vi "Navigation_Main_derping_stuff_up 5th.vi"() -> ()   [LabVIEW 2015]
uses:
  <vilib>/myRIO/Common/Instrument Driver Framework/Utilities/typedefs/Generic FPGA Reference.ctl
  <vilib>/myRIO/Common/Instrument Driver Framework/Utilities/typedefs/myRIO v1.0 Reference.ctl
  <vilib>/myRIO/Common/Instrument Driver Framework/Utilities/typedefs/Hardware Version Enum.ctl
  <vilib>/myRIO/Common/Instrument Driver Framework/Utilities/typedefs/myRIO Generic Hardware Reference.ctl
  <vilib>/userdefined/High Color/nirio_resource_hc.ctl
  <vilib>/myRIO/Instrument Drivers/Onboard IO/PWM/typedefs/PWM Configuration.ctl
  <vilib>/myRIO/Instrument Drivers/Onboard IO/PWM/PWM.lvlib
  <vilib>/myRIO/Common/Instrument Driver Framework/myRIO v1.0/PWM/typedefs/PWM Channels Enum.ctl
  <vilib>/myRIO/Instrument Drivers/Onboard IO/PWM/typedefs/PWM Reference.ctl
  <vilib>/myRIO/Instrument Drivers/Onboard IO/PWM/vis/myRIO PWM Open.xnode
  <vilib>/myRIO/Common/Instrument Driver Framework/myRIO v1.0/PWM/vis/myRIO v1.1 Open PWM.vi
  <vilib>/rvi/interface/nirviOpenFPGA/nirviOpenFPGA.xnode
  <vilib>/myRIO/Instrument Drivers/Utilities/Utilities.lvlib
  <vilib>/rvi/interface/nirviReadWriteControl/nirviReadWriteControl.xnode
  <vilib>/rvi/interface/Simulation/niFpgaSimulationCallBeginRW.vi
  <vilib>/rvi/errors/niLvFpgaAdjustHostInterfaceError.vi
  UNCC_AST2_Master/FPGA Bitfiles/NavigationProjec_FPGATarget2_FPGAMainNavigati_PWPHW8gwDxI.lvbitx
  <vilib>/addons/control/pid/NI_PID_pid.lvlib
  <vilib>/addons/control/pid/pid.llb/PID (DBL).vi
  <vilib>/FPGAPlugInAG/myRIO-1900/niLvFpga_Open_myRIO-1900.vi
  <vilib>/rvi/interface/common/dynamic/niFpgaDynamicAddResources.vi
panel:
  out "x/y":dbl
  out "scale":dbl=1.0
  in  "x goal":dbl=20.0
  out "left":dbl
  out "right":dbl
  out "actual pwm left":dbl
  in  "stop 3":bool
  out "left pwm":dbl(graph)
  out "dt out (s) left":dbl format="%.3f"
  in  "output range 3":cluster{"output high":dbl, "output low":dbl}={"output high"=0.13333, "output low"=-0.13333} {"output low" format="%.6f"; "output high" format="%.5f"}
  in  "PID gains 3":T1={"proportional gain (Kc)"=0.002, "integral time (Ti, min)"=7e-07, "derivative time (Td, min)"=0.0} {"derivative time (Td, min)" format="%.8f"; "integral time (Ti, min)" format="%.8f"; "proportional gain (Kc)" format="%.8f"}
  out "desired pwm 2":dbl
  out "feedback 2":dbl
  out ".not. x? 3":bool
  out "Elapsed Time (s) 2":dbl caption="Elapsed Time (s)"
  out "x traveled 2":dbl
  out "y traveled 2":dbl
  out "avg 124":dbl
  out "avg 457":dbl
  out "psi dot 2":dbl
  out "distance traveled 2":dbl
  out "y dot 2":dbl
  out "x dot 2":dbl
  out "x position 2":dbl
  out "y position 2":dbl
  out "reset x y 2":dbl
  out "Tick Count(mSec) 2":u32 caption="Tick Count(mSec)"
  in  "start y 2":dbl=3.0
  in  "start x 2":dbl=1.0
  in  "start y":dbl=3.0
  in  "start x":dbl=1.0
  out "actual pwm right":dbl
  in  "stop 2":bool
  out "right pwm":dbl(graph)
  out "dt out (s) right":dbl format="%.3f"
  in  "output range 2":cluster{"output high":dbl, "output low":dbl}={"output high"=0.13333, "output low"=-0.13333} {"output low" format="%.6f"; "output high" format="%.5f"}
  in  "PID gains 2":T1={"proportional gain (Kc)"=0.002, "integral time (Ti, min)"=7e-07, "derivative time (Td, min)"=0.0} {"derivative time (Td, min)" format="%.8f"; "integral time (Ti, min)" format="%.8f"; "proportional gain (Kc)" format="%.8f"}
  out "desired pwm":dbl
  out "feedback right":dbl
  out ".not. x? 2":bool
  out "Elapsed Time (s)":dbl
  out "LF Rot Velocity (rot/s)":dbl
  out "LM Rot Velocity (rot/s)":dbl
  out "LR Rot Velocity (rot/s)":dbl
  out "RR Rot Velocity (rot/s)":dbl
  out "RM Linear Velocity (rot/s)":dbl
  out "RF Linear Velocity (rot/s)":dbl
  in  "Encoder Reset":bool
  out "SYS.SELECTA":u8 format="%08b"
  out "ENC.B_c.CNTR":i32
  out "ENC.B_b.CNTR":i32
  out "ENC.B_a.CNTR":i32
  out "ENC.A_c.CNTR":i32
  out "ENC.A_b.CNTR":i32
  out "ENC.A_a.CNTR":i32
  in  "R Min Linear Velocity (ft/s)":dbl=-2.0 format="%#_13g"
  in  "R Max Linear Velocity (ft/s)":dbl=2.0 format="%#_13g"
  in  "L Min Linear Velocity (ft/s)":dbl=-2.0 format="%#_13g"
  in  "L Max Linear Velocity (ft/s)":dbl=2.0 format="%#_13g"
  out "Current Rot Velocity (rot/s)":T2(graph)
  # "Motor Control Parameters"
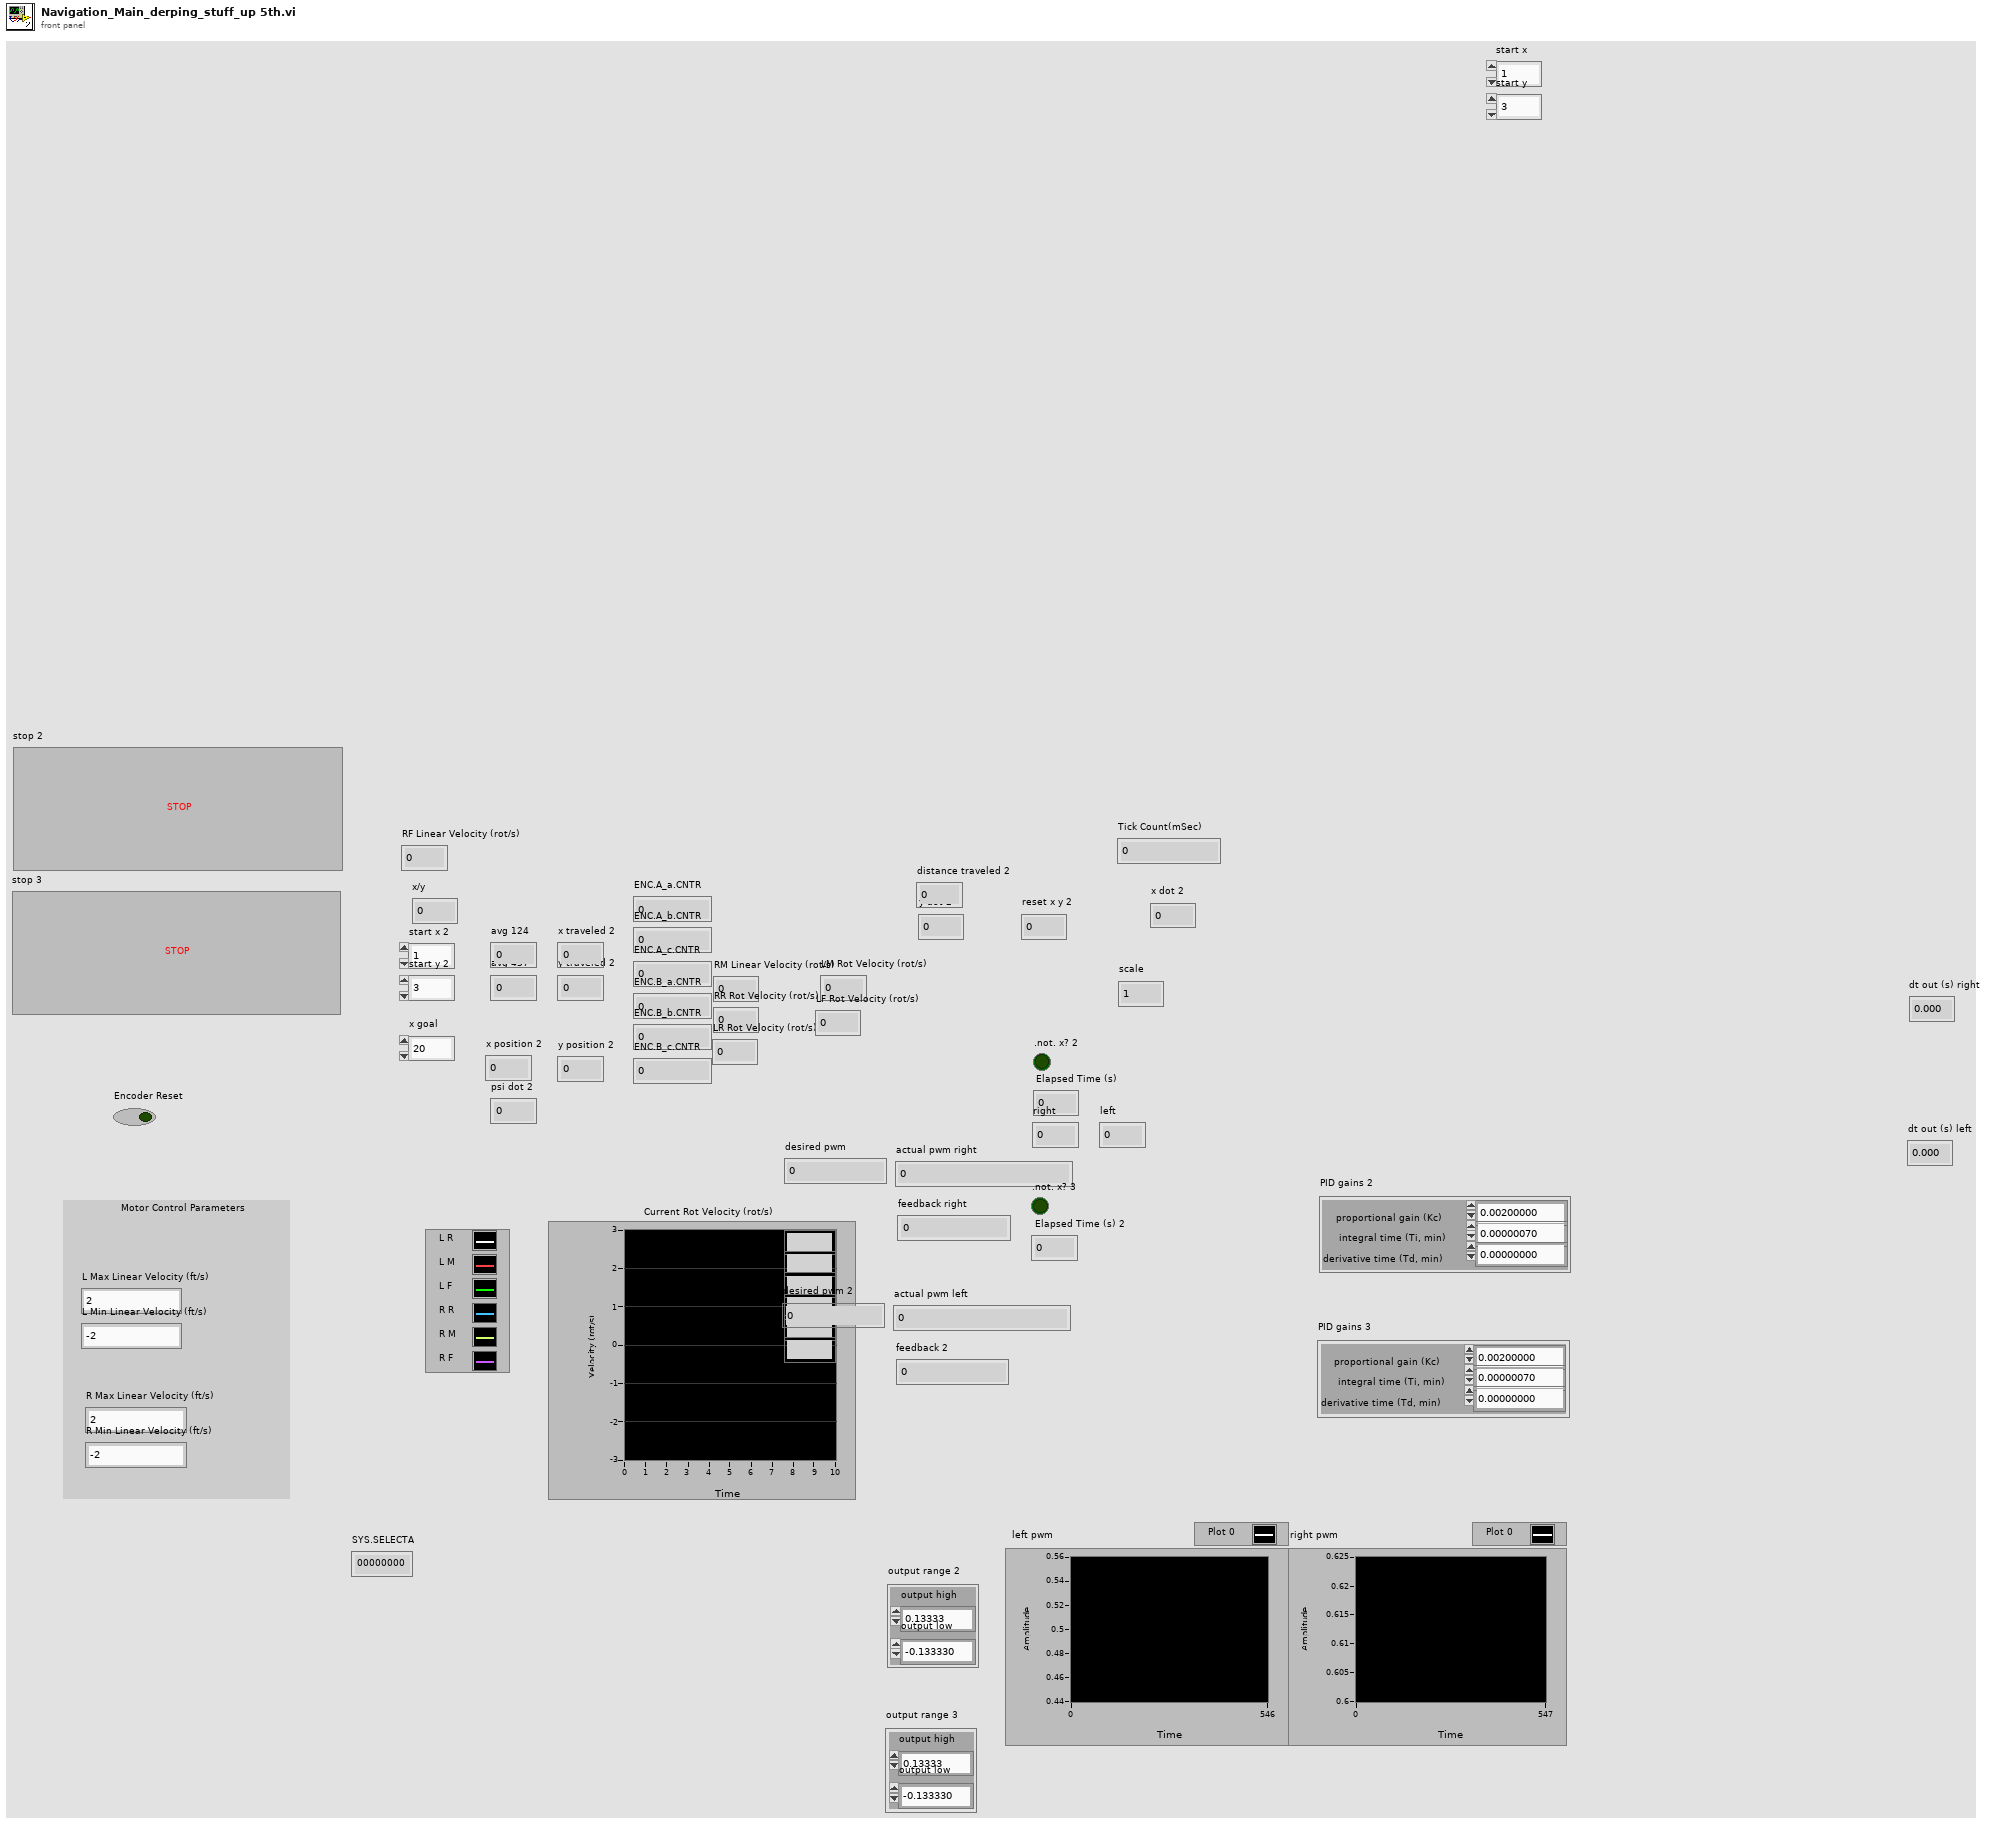
[diagram p1: front panel]
types:
  T1 = cluster{"proportional gain (Kc)":dbl, "integral time (Ti, min)":dbl, "derivative time (Td, min)":dbl}
  T2 = cluster{"Rotational Velocity (RPS)":dbl, "Rotational Velocity (RPS)":dbl, "Rotational Velocity (RPS)":dbl, "Rotational Velocity (RPS)":dbl, "Rotational Velocity (RPS)":dbl, "Rotational Velocity (RPS)":dbl}
  T3 = typedef "nirio_resource_hc.ctl" = tag
  T4 = typedef "Hardware Version Enum.ctl" = enum16{"Unknown", "myRIO-1900", "myRIO-1950", "roboRIO"}
  T5 = typedef "PWM.lvlib/PWM Reference.ctl" = cluster{"myRIO Reference":T6, "PWM Channels Enum":T9, "PWM Configuration":T10}
  T6 = typedef "myRIO Generic Hardware Reference.ctl" = cluster{"myRIO Model":T4, "myRIO Hardware Reference":T7}
  T7 = typedef "myRIO v1.0 Reference.ctl" = cluster{"Generic FPGA Reference":T8, "Allow multiple opens":bool}
  T8 = typedef "Generic FPGA Reference.ctl" = refnum<k20>
  T9 = typedef "PWM Channels Enum.ctl" = enum16{"Not Connected", "C/PWM0", "C/PWM1", "A/PWM0", "A/PWM1", "A/PWM2", "B/PWM0", "B/PWM1", "B/PWM2", "PWM/PWM0", "PWM/PWM1", "PWM/PWM2", "PWM/PWM3", "PWM/PWM4", "PWM/PWM5", "PWM/PWM6", "PWM/PWM7", "PWM/PWM8", "PWM/PWM9"}
  T10 = typedef "PWM.lvlib/PWM Configuration.ctl" = cluster{"Frequency":dbl, "Duty Cycle":dbl}
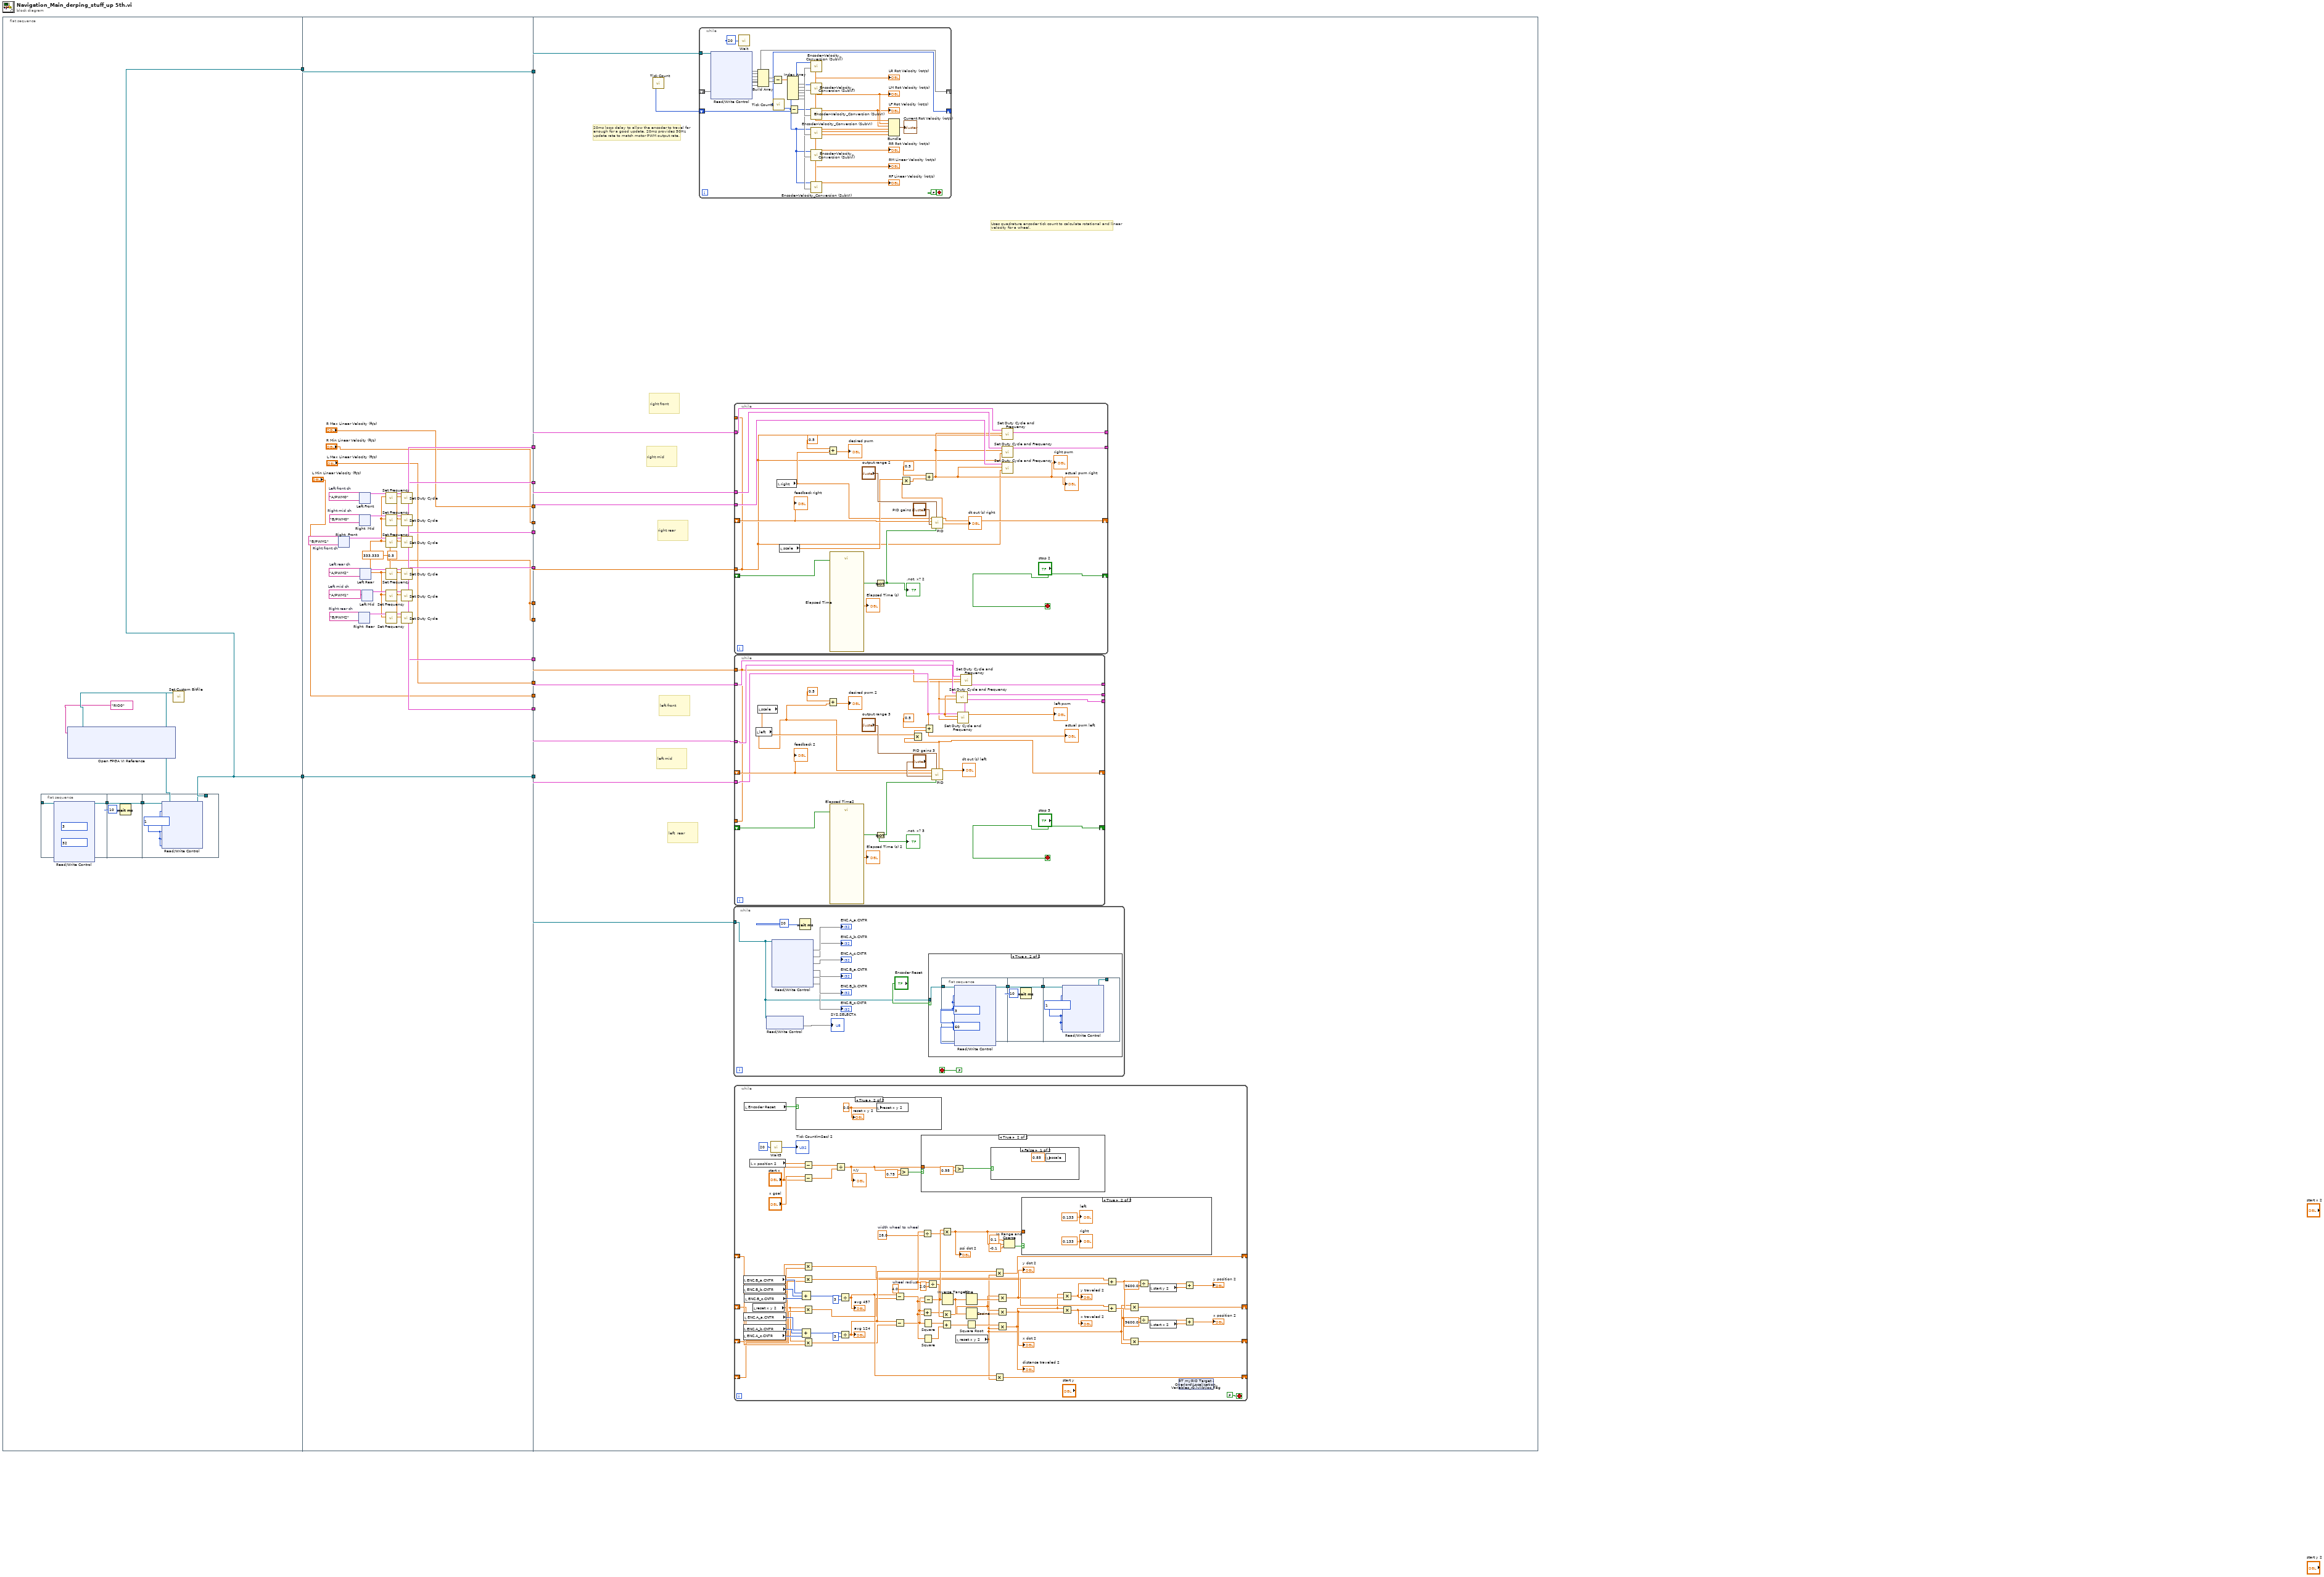
[diagram p0: block diagram]
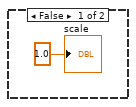
[diagram p2: hidden frame]
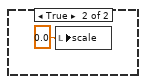
[diagram p3: hidden frame]
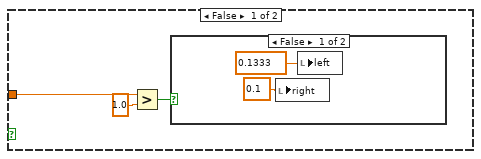
[diagram p4: hidden frame]
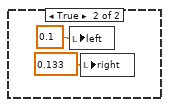
[diagram p5: hidden frame]
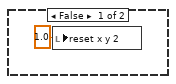
[diagram p6: hidden frame]
diagram:
  n1 = flat-sequence {
    tunnel: [w19] -> w4
    tunnel: [w19] -> w2
    tunnel: [w32] -> w16
    tunnel: [w47] -> w15
    tunnel: [w43] -> w14
    tunnel: [w42] -> w13
    tunnel: [w41] -> w12
    tunnel: [w40] -> w11
    tunnel: [w39] -> w10
    tunnel: ["L Max Linear Velocity (ft/s)"] -> w9
    tunnel: ["L Min Linear Velocity (ft/s)"] -> w8
    tunnel: ["R Max Linear Velocity (ft/s)"] -> w7
    tunnel: ["R Min Linear Velocity (ft/s)"] -> w6
    tunnel: [w34] -> w5
    tunnel: w4 -> [w33]
    tunnel: [w33] -> w3
    tunnel: w2 -> [w34]
    tunnel: [w32] -> w1
    tunnel: w16 -> [_]
    tunnel: w15 -> [w160]
    tunnel: w14 -> [w166]
    tunnel: w13 -> [w162]
    tunnel: w12 -> [w163]
    tunnel: w11 -> [w161]
    tunnel: w10 -> [w165]
    tunnel: w9 -> [_]
    tunnel: w8 -> [_]
    tunnel: w7 -> [_]
    tunnel: w6 -> [_]
    tunnel: w5 -> [w168]
    tunnel: w3 -> [w167]
    tunnel: w1 -> [w164]
    frame #0 {
      n2 = flat-sequence {
        tunnel: w20 -> [w25]
        tunnel: [w23] -> w22
        tunnel: w22 -> [w27]
        tunnel: [w27] -> w21
        tunnel: w21 -> [w30]
        tunnel: [w29] -> w19
        frame #0 {
          w24 = u8 32 ("SYS.SELECTA")
          w26 = u8 3 ("ENC.B_c.CNFG")
          n3 = xnode "Read/Write Control"("FPGA VI Reference In"=w25, "ENC.A_a.CNFG"=w26, "ENC.A_b.CNFG"=w26, "ENC.A_c.CNFG"=w26, "ENC.B_a.CNFG"=w26, "ENC.B_b.CNFG"=w26, "ENC.B_c.CNFG"=w26, "SYS.SELECTA"=w24, "SYS.SELECTB"=w24) -> ("FPGA VI Reference Out"=w23:refnum<k20>)  [unwired: 1 in, 1 out]
        }
        frame #1 {
          n4 = Wait (ms)(milliseconds to wait=u32 10) -> ()  [unwired: 1 out]
        }
        frame #2 {
          w31 = u8 1 ("ENC.B_c.CNFG")
          n5 = xnode "Read/Write Control"("FPGA VI Reference In"=w30, "ENC.A_a.CNFG"=w31, "ENC.A_b.CNFG"=w31, "ENC.A_c.CNFG"=w31, "ENC.B_a.CNFG"=w31, "ENC.B_b.CNFG"=w31, "ENC.B_c.CNFG"=w31) -> ("FPGA VI Reference Out"=w29:refnum<k20>)  [unwired: 1 in, 1 out]
        }
      }
      n6 = xnode "Open FPGA VI Reference"("resource name"=tag "RIO0") -> ("FPGA VI Reference Out"=w18:refnum<k20>)  [unwired: 1 in, 1 out]
      n7 = call <vilib>:"Set Custom Bitfile.vi"("Custom FPGA Reference In"=w18) -> ("Custom FPGA Reference Out"=w20:refnum<k20>)  [unwired: 9 in, 1 out]
    }
    frame #1 {
      w44 = 0.5 ("Duty Cycle")
      w32 = 333.333 ("Frequency [Hz]")
      w58 = tag "B/PWM2"  # Right rear ch
      w59 = tag "B/PWM0"  # Right mid ch
      w60 = tag "B/PWM1"  # Right front ch
      w61 = tag "A/PWM2"  # Left rear ch
      w62 = tag "A/PWM1"  # Left mid ch
      w63 = tag "A/PWM0"  # Left front ch
      n8 = xnode "Right  Front"("Channel Name"=w60) -> ("PWM Ref Out"=w54:T5)  [unwired: 2 in, 1 out]
      n9 = xnode "Right  Rear"("Channel Name"=w58) -> ("PWM Ref Out"=w52:T5)  [unwired: 2 in, 1 out]
      n10 = xnode "Left Front"("Channel Name"=w63) -> ("PWM Ref Out"=w57:T5)  [unwired: 2 in, 1 out]
      n11 = xnode "Right  Mid"("Channel Name"=w59) -> ("PWM Ref Out"=w53:T5)  [unwired: 2 in, 1 out]
      n12 = xnode "Left Rear"("Channel Name"=w61) -> ("PWM Ref Out"=w55:T5)  [unwired: 2 in, 1 out]
      n13 = xnode "Left Mid"("Channel Name"=w62) -> ("PWM Ref Out"=w56:T5)  [unwired: 2 in, 1 out]
      n14 = call <vilib>:"Set Frequency.vi"("Frequency [Hz]"=w32, "PWM Ref In"=w57) -> ("PWM Ref Out"=w51:T5)  [unwired: 7 in, 1 out]
      n15 = call <vilib>:"Set Frequency.vi"("Frequency [Hz]"=w32, "PWM Ref In"=w53) -> ("PWM Ref Out"=w49:T5)  [unwired: 7 in, 1 out]
      n16 = call <vilib>:"Set Frequency.vi"("Frequency [Hz]"=w32, "PWM Ref In"=w54) -> ("PWM Ref Out"=w48:T5)  [unwired: 7 in, 1 out]
      n17 = call <vilib>:"Set Frequency.vi"("Frequency [Hz]"=w32, "PWM Ref In"=w55) -> ("PWM Ref Out"=w46:T5)  [unwired: 7 in, 1 out]
      n18 = call <vilib>:"Set Frequency.vi"("Frequency [Hz]"=w32, "PWM Ref In"=w56) -> ("PWM Ref Out"=w45:T5)  [unwired: 7 in, 1 out]
      n19 = call <vilib>:"Set Frequency.vi"("Frequency [Hz]"=w32, "PWM Ref In"=w52) -> ("PWM Ref Out"=w50:T5)  [unwired: 7 in, 1 out]
      n20 = call <vilib>:"Set Duty Cycle.vi"("Duty Cycle"=w44, "PWM Ref In"=w51) -> ("PWM Ref Out"=w39:T5)  [unwired: 7 in, 1 out]
      n21 = call <vilib>:"Set Duty Cycle.vi"("Duty Cycle"=w44, "PWM Ref In"=w49) -> ("PWM Ref Out"=w42:T5)  [unwired: 7 in, 1 out]
      n22 = call <vilib>:"Set Duty Cycle.vi"("Duty Cycle"=w44, "PWM Ref In"=w48) -> ("PWM Ref Out"=w43:T5)  [unwired: 7 in, 1 out]
      n23 = call <vilib>:"Set Duty Cycle.vi"("Duty Cycle"=w44, "PWM Ref In"=w46) -> ("PWM Ref Out"=w47:T5)  [unwired: 7 in, 1 out]
      n24 = call <vilib>:"Set Duty Cycle.vi"("Duty Cycle"=w44, "PWM Ref In"=w45) -> ("PWM Ref Out"=w40:T5)  [unwired: 7 in, 1 out]
      n25 = call <vilib>:"Set Duty Cycle.vi"("Duty Cycle"=w44, "PWM Ref In"=w50) -> ("PWM Ref Out"=w41:T5)  [unwired: 7 in, 1 out]
    }
    frame #2 {
      # "left  rear"
      # "left mid"
      # "left front"
      # "right rear"
      # "right mid"
      # "right front"
      # "Uses quadrature encoder tick count to calculate rotational and linear velocity for a wheel."
      # "20ms loop delay to allow the encoder to travel far enough for a good update. 20ms provides 50Hz update rate to match motor PWM output rate."
      n26 = call "Tick Count"() -> ("Tick Count(uSec)"=w169:u32)
      n27 = while {
        shift-right: [w349] -> _
        shift-left: _ -> [w348]
        shift-right: [w346] -> _
        shift-left: w169 -> [w345]
        tunnel: w167 -> [w356]
        stop <- FALSE stop-if-true
        n28 = xnode "Read/Write Control"("FPGA VI Reference In"=w356) -> ("ENC.A_a.CNTR"=w355, "ENC.A_b.CNTR"=w354, "ENC.A_c.CNTR"=w353, "ENC.B_a.CNTR"=w352, "ENC.B_b.CNTR"=w351, "ENC.B_c.CNTR"=w350)  [unwired: 1 in, 2 out]
        n29 = call "Wait"("Count(mSec)"=u32 20) -> ()  [unwired: 1 out]
        n30 = Build Array(w355, w354, w353, w352, w351, w350) -> (w349:void[])
        n31 = Subtract(x=w349, y=w348) -> (x-y=w347:dbl)
        n32 = call "Tick Count2"() -> ("Tick Count(uSec)"=w346:u32)
        n33 = Index Array(array=w347) -> (element #1=w344, element #2=w343, element #3=w342, element #4=w341, element #5=w340, element #6=w339)  [unwired: 6 in]
        n34 = Subtract(x=w346, y=w345) -> (x-y=w338:u32)
        n35 = call "Encoder-Velocity_Conversion (SubVI).vi"("delta  Encoder Count"=w343, "dt (uSec)"=w338) -> ("Rotational Velocity (RPS)"=w333:dbl)  [unwired: 7 in, 2 out]
        "LM Rot Velocity (rot/s)" <- w333
        n36 = call "Encoder-Velocity_Conversion (SubVI).vi"("delta  Encoder Count"=w342, "dt (uSec)"=w338) -> ("Rotational Velocity (RPS)"=w332:dbl)  [unwired: 7 in, 2 out]
        "LF Rot Velocity (rot/s)" <- w332
        n37 = call "Encoder-Velocity_Conversion (SubVI).vi"("delta  Encoder Count"=w344, "dt (uSec)"=w338) -> ("Rotational Velocity (RPS)"=w334:dbl)  [unwired: 7 in, 2 out]
        "LR Rot Velocity (rot/s)" <- w334
        n38 = call "Encoder-Velocity_Conversion (SubVI).vi"("delta  Encoder Count"=w341, "dt (uSec)"=w338) -> ("Rotational Velocity (RPS)"=w331:dbl)  [unwired: 7 in, 2 out]
        "RR Rot Velocity (rot/s)" <- w331
        n39 = call "Encoder-Velocity_Conversion (SubVI).vi"("delta  Encoder Count"=w340, "dt (uSec)"=w338) -> ("Rotational Velocity (RPS)"=w335:dbl)  [unwired: 7 in, 2 out]
        "RM Linear Velocity (rot/s)" <- w335
        n40 = call "Encoder-Velocity_Conversion (SubVI).vi"("delta  Encoder Count"=w339, "dt (uSec)"=w338) -> ("Rotational Velocity (RPS)"=w336:dbl)  [unwired: 7 in, 2 out]
        "RF Linear Velocity (rot/s)" <- w336
        n41 = Bundle("Rotational Velocity (RPS)"=w334, "Rotational Velocity (RPS)"=w333, "Rotational Velocity (RPS)"=w332, "Rotational Velocity (RPS)"=w331, "Rotational Velocity (RPS)"=w335, "Rotational Velocity (RPS)"=w336) -> (→"Current Rot Velocity (rot/s)":T2)  [unwired: 1 in]
      }
      n42 = while {
        tunnel: w168 -> [w308]
        stop <- FALSE stop-if-true
        n43 = xnode "Read/Write Control"("FPGA VI Reference In"=w308) -> ("SYS.SELECTA"=→"SYS.SELECTA")  [unwired: 1 in, 2 out]
        n44 = xnode "Read/Write Control"("FPGA VI Reference In"=w308) -> ("ENC.A_a.CNTR"=→"ENC.A_a.CNTR", "ENC.A_b.CNTR"=→"ENC.A_b.CNTR", "ENC.A_c.CNTR"=→"ENC.A_c.CNTR", "ENC.B_a.CNTR"=→"ENC.B_a.CNTR", "ENC.B_b.CNTR"=→"ENC.B_b.CNTR", "ENC.B_c.CNTR"=→"ENC.B_c.CNTR")  [unwired: 1 in, 2 out]
        n45 = Wait (ms)(milliseconds to wait=u32 20) -> ()  [unwired: 1 out]
        n46 = case shown="True" "Encoder Reset" {
          tunnel: w308 -> [_ w319]
          frame False {
          }
          frame True {
            n47 = flat-sequence {
              tunnel: w319 -> [w324]
              tunnel: [w322] -> w321
              tunnel: w321 -> [w326]
              tunnel: [w326] -> w320
              tunnel: w320 -> [w329]
              tunnel: [w328] -> _
              frame #0 {
                w323 = u8 60 ("SYS.SELECTA")
                w325 = u8 3 ("ENC.B_c.CNFG")
                n48 = xnode "Read/Write Control"("FPGA VI Reference In"=w324, "ENC.A_a.CNFG"=w325, "ENC.A_b.CNFG"=w325, "ENC.A_c.CNFG"=w325, "ENC.B_a.CNFG"=w325, "ENC.B_b.CNFG"=w325, "ENC.B_c.CNFG"=w325, "SYS.SELECTA"=w323, "SYS.SELECTB"=w323) -> ("FPGA VI Reference Out"=w322:refnum<k20>)  [unwired: 1 in, 1 out]
              }
              frame #1 {
                n49 = Wait (ms)(milliseconds to wait=u32 10) -> ()  [unwired: 1 out]
              }
              frame #2 {
                w330 = u8 1 ("ENC.B_c.CNFG")
                n50 = xnode "Read/Write Control"("FPGA VI Reference In"=w329, "ENC.A_a.CNFG"=w330, "ENC.A_b.CNFG"=w330, "ENC.A_c.CNFG"=w330, "ENC.B_a.CNFG"=w330, "ENC.B_b.CNFG"=w330, "ENC.B_c.CNFG"=w330) -> ("FPGA VI Reference Out"=w328:refnum<k20>)  [unwired: 1 in, 1 out]
              }
            }
          }
        }
      }
      n51 = while {
        tunnel: w166 -> [w306]
        tunnel: [w307] -> _
        tunnel: [w285] -> _
        shift-right: [w292] -> _
        shift-left: _ -> [w302]
        shift-right: ["stop 2"] -> _
        shift-left: _ -> [w297]
        tunnel: w164 -> [w285]
        tunnel: w163 -> [w287]
        tunnel: w162 -> [w289]
        tunnel: [w288] -> _
        stop <- "stop 2" stop-if-true
        n52 = local read "right"() -> (w290:dbl)
        n53 = local read "scale"() -> (w293:dbl)
        n54 = Add(x=0.5, y=w290) -> (x+y=→"desired pwm":dbl)
        n55 = call "Elapsed Time"("Reset"=w297) -> ("Elapsed Time (s)"=→"Elapsed Time (s)":dbl, "Time has Elapsed"=w300:bool)  [unwired: 11 in, 6 out]
        n56 = Not(x=w300) -> (.not. x?=w299:bool)
        ".not. x? 2" <- w299
        n57 = call-poly <vilib>:"PID.vi"("reinitialize? (F)"=w299, "output range"="output range 2", "PID gains"="PID gains 2", "process variable"=w302, "setpoint"=w290) -> ("dt out (s)"=→"dt out (s) right":dbl, "output"=w292:dbl)  [unwired: 5 in]
        n58 = Multiply(x=w293, y=w292) -> (x*y=w291:dbl)
        n59 = Add(x=0.5, y=w291) -> (x+y=w286:dbl)
        "actual pwm right" <- w286
        "right pwm" <- w286
        n60 = call <vilib>:"Set Duty Cycle and Frequency.vi"("Frequency [Hz]"=w285, "Duty Cycle"=w286, "PWM Ref In"=w306) -> ("PWM Ref Out"=w307:T5)  [unwired: 6 in, 1 out]
        n61 = call <vilib>:"Set Duty Cycle and Frequency.vi"("Frequency [Hz]"=w285, "Duty Cycle"=w286, "PWM Ref In"=w289) -> ("PWM Ref Out"=w288:T5)  [unwired: 6 in, 1 out]
        n62 = call <vilib>:"Set Duty Cycle and Frequency.vi"("Frequency [Hz]"=w285, "Duty Cycle"=w286, "PWM Ref In"=w287) -> ()  [unwired: 6 in, 2 out]
        "feedback right" <- w302
      }
      n63 = while {
        tunnel: w165 -> [w192]
        tunnel: [w193] -> _
        tunnel: w164 -> [w172]
        shift-right: [w178] -> _
        shift-left: _ -> [w188]
        shift-right: ["stop 3"] -> _
        shift-left: _ -> [w183]
        tunnel: [w172] -> _
        tunnel: w161 -> [w175]
        tunnel: w160 -> [w174]
        tunnel: [w171] -> _
        tunnel: [w170] -> _
        stop <- "stop 3" stop-if-true
        n64 = local read "left"() -> (w176:dbl)
        n65 = local read "scale"() -> (w179:dbl)
        n66 = Add(x=0.5, y=w176) -> (x+y=→"desired pwm 2":dbl)
        n67 = call "Elapsed Time2"("Reset"=w183) -> ("Elapsed Time (s)"=→"Elapsed Time (s) 2":dbl, "Time has Elapsed"=w186:bool)  [unwired: 11 in, 6 out]
        n68 = Not(x=w186) -> (.not. x?=w185:bool)
        ".not. x? 3" <- w185
        n69 = call-poly <vilib>:"PID.vi"("reinitialize? (F)"=w185, "output range"="output range 3", "PID gains"="PID gains 3", "process variable"=w188, "setpoint"=w176) -> ("dt out (s)"=→"dt out (s) left":dbl, "output"=w178:dbl)  [unwired: 5 in]
        n70 = Multiply(x=w179, y=w178) -> (x*y=w177:dbl)
        n71 = Add(x=0.5, y=w177) -> (x+y=w173:dbl)
        "actual pwm left" <- w173
        "left pwm" <- w173
        n72 = call <vilib>:"Set Duty Cycle and Frequency.vi"("Frequency [Hz]"=w172, "Duty Cycle"=w173, "PWM Ref In"=w175) -> ("PWM Ref Out"=w171:T5)  [unwired: 6 in, 1 out]
        n73 = call <vilib>:"Set Duty Cycle and Frequency.vi"("Frequency [Hz]"=w172, "Duty Cycle"=w173, "PWM Ref In"=w174) -> ("PWM Ref Out"=w170:T5)  [unwired: 6 in, 1 out]
        n74 = call <vilib>:"Set Duty Cycle and Frequency.vi"("Frequency [Hz]"=w172, "Duty Cycle"=w173, "PWM Ref In"=w192) -> ("PWM Ref Out"=w193:T5)  [unwired: 6 in, 1 out]
        "feedback 2" <- w188
      }
      n75 = while {
        shift-right: [w216] -> _
        shift-left: _ -> [w254]
        shift-right: [w213] -> _
        shift-left: _ -> [w253]
        shift-right: [w215] -> _
        shift-left: _ -> [w228]
        shift-right: [w214] -> _
        shift-left: _ -> [w227]
        stop <- FALSE stop-if-true
        w249 = 28.0  # width wheel to wheel
        w250 = 4.0  # wheel radius
        n76 = local read "ENC.B_a.CNTR"() -> (w259:i32)
        n77 = local read "ENC.B_b.CNTR"() -> (w258:i32)
        n78 = local read "ENC.A_b.CNTR"() -> (w261:i32)
        n79 = local read "ENC.A_c.CNTR"() -> (w260:i32)
        n80 = local read "ENC.A_a.CNTR"() -> (w262:i32)
        n81 = local read "Encoder Reset"() -> (w209:bool)
        n82 = local read "ENC.B_c.CNTR"() -> (w257:i32)
        n83 = local read "x position 2"() -> (w201:dbl)
        n84 = local read "reset x y 2"() -> (w212:dbl)
        n85 = call "Wait3"("Count(mSec)"=u32 20) -> ("Tick Count(mSec)"=→"Tick Count(mSec) 2":u32)
        n86 = case shown="True" w209 {
          frame False {
            n87 = local write "reset x y 2"(1.0) -> ()
          }
          frame True {
            w284 = 0.0
            n88 = local write "reset x y 2"(w284) -> ()
            "reset x y 2" <- w284
          }
        }
        n89 = Compound Arithmetic op=ADD(w259, w258, w257) -> (w265:i32)
        n90 = Compound Arithmetic op=ADD(w262, w261, w260) -> (w266:i32)
        n91 = Subtract(x=w201, y="start x") -> (x-y=w195:dbl)
        n92 = Subtract(x="x goal", y="start x") -> (x-y=w194:dbl)
        n93 = Multiply(x=w212, y=w228) -> (x*y=w219:dbl)
        n94 = Multiply(x=w212, y=w227) -> (x*y=w218:dbl)
        n95 = Multiply(x=w212, y=w253) -> (x*y=w217:dbl)
        n96 = Multiply(x=w212, y=w254) -> (x*y=w220:dbl)
        n97 = Divide(x=w195, y=w194) -> (x/y=w198:dbl)
        "x/y" <- w198
        n98 = Divide(x=w265, y=3) -> (x/y=w252:dbl)
        "avg 457" <- w252
        n99 = Divide(x=w266, y=3) -> (x/y=w255:dbl)
        "avg 124" <- w255
        n100 = Subtract(x=w252, y=w217) -> (x-y=w242:dbl)
        n101 = Subtract(x=w255, y=w220) -> (x-y=w243:dbl)
        n102 = Greater?(x=w198, y=0.75) -> (0:w199:bool)
        n103 = case shown="True" w199 {
          tunnel: w198 -> [_ w271]
          frame False {
            "scale" <- 1.0
          }
          frame True {
            n104 = Greater?(x=w271, y=0.95) -> (0:w269:bool)
            n105 = case shown="False" w269 {
              frame False {
                n106 = local write "scale"(0.85) -> ()
              }
              frame True {
                n107 = local write "scale"(0.0) -> ()
              }
            }
          }
        }
        n108 = Divide(x=w250, y=w249) -> (x/y=w245:dbl)
        n109 = Add(x=w243, y=w242) -> (x+y=w247:dbl)
        n110 = Square(x=w243) -> (x^2=w240:dbl)
        n111 = Square(x=w242) -> (x^2=w241:dbl)
        n112 = Subtract(x=w243, y=w242) -> (x-y=w246:dbl)
        n113 = Divide(x=w250, y=2.0) -> (x/y=w248:dbl)
        n114 = Multiply(x=w247, y=w248) -> (x*y=w236:dbl)
        n115 = Add(x=w240, y=w241) -> (x+y=w239:dbl)
        n116 = Multiply(x=w246, y=w245) -> (x*y=w202:dbl)
        "psi dot 2" <- w202
        n117 = Inverse Tangent(1:w246) -> (0:w244:dbl)
        n118 = local read "reset x y 2"() -> (w210:dbl)
        n119 = Square Root(x=w239) -> (sqrt(x)=w233:dbl)
        n120 = Sine(x=w244) -> (sin(x)=w238:dbl)
        n121 = Cosine(x=w244) -> (cos(x)=w237:dbl)
        n122 = Multiply(x=w255, y=w210) -> (x*y=w216:dbl)
        n123 = Multiply(x=w252, y=w210) -> (x*y=w213:dbl)
        n124 = Multiply(x=w236, y=w238) -> (x*y=w235:dbl)
        "y dot 2" <- w235
        n125 = Multiply(x=w236, y=w237) -> (x*y=w234:dbl)
        "x dot 2" <- w234
        n126 = Multiply(x=w233, y=w210) -> (x*y=w211:dbl)
        "distance traveled 2" <- w211
        n127 = In Range and Coerce(upper limit=0.1, x=w202, lower limit=-0.1) -> (In Range?=w203:bool)  [unwired: 1 out]
        n128 = case shown="True" w203 {
          tunnel: w202 -> [w276 _]
          frame False {
            n129 = Greater?(x=w276, y=1.0) -> (0:w274:bool)
            n130 = case shown="False" w274 {
              frame False {
                n131 = local write "right"(0.1) -> ()
                n132 = local write "left"(0.1333) -> ()
              }
              frame True {
                n133 = local write "left"(0.1) -> ()
                n134 = local write "right"(0.133) -> ()
              }
            }
          }
          frame True {
            "right" <- 0.133
            "left" <- 0.133
          }
        }
        n135 = Multiply(x=w211, y=w235) -> (x*y=w231:dbl)
        "y traveled 2" <- w231
        n136 = Multiply(x=w211, y=w234) -> (x*y=w232:dbl)
        "x traveled 2" <- w232
        n137 = Add(x=w219, y=w231) -> (x+y=w222:dbl)
        n138 = Add(x=w218, y=w232) -> (x+y=w230:dbl)
        n139 = Multiply(x=w210, y=w222) -> (x*y=w215:dbl)
        n140 = Multiply(x=w230, y=w210) -> (x*y=w214:dbl)
        n141 = Divide(x=w222, y=9600.0) -> (x/y=w226:dbl)
        n142 = Divide(x=w230, y=9600.0) -> (x/y=w225:dbl)
        n143 = local read "start y 2"() -> (w224:dbl)
        n144 = local read "start x 2"() -> (w223:dbl)
        n145 = shared-variable "RT myRIO Target - Overlord\\Localization_Variables_r0.lvlib\\loc_flag"() -> ()  [unwired: 1 in, 2 out]
        n146 = Add(x=w226, y=w224) -> (x+y=→"y position 2":dbl)
        n147 = Add(x=w225, y=w223) -> (x+y=→"x position 2":dbl)
      }
    }
  }
